vi "Constants.vi"   [LabVIEW 2017, in "Data Sharing Framework Core.lvlib" / "Data Sharing Framework Engine.lvlib"]
uses:
  Data Sharing Framework Engine.lvlib
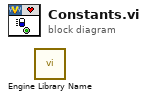
[diagram p0: block diagram]
diagram:
  n1 = call "Engine Library Name.vi"() -> ()  [unwired: 11 in, 1 out]
